vi "Wii_2D_mapping.vi"(0 "Wii_X_off":dbl, 5 "Wii_Y_off":dbl, 9 "previous_X":i32, 11 "previous_Y":i32, 13 "X_Y_speed":dbl) -> (4 "X":i32, 6 "Y":i32)   [LabVIEW 2011]
panel:
  out "X_resolution":i16
  out "Y_resolution":i16
  out "Ymax":i16
  out "Xmax":i16=2
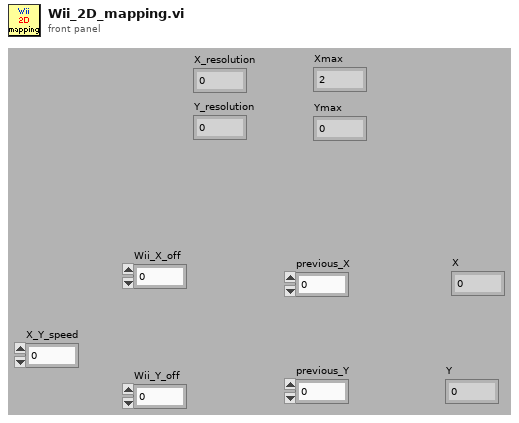
[diagram p1: front panel]
types:
  T1 = typedef "LVAllMonitorsDisplayTypeDef.ctl" = cluster{"Bounds":cluster{"Left":i16, "Top":i16, "Right":i16, "Bottom":i16}, "Depth":i16}[]
  T2 = cluster{"Bounds":cluster{"Left":i16, "Top":i16, "Right":i16, "Bottom":i16}, "Depth":i16}
  T3 = cluster{"Left":i16, "Top":i16, "Right":i16, "Bottom":i16}
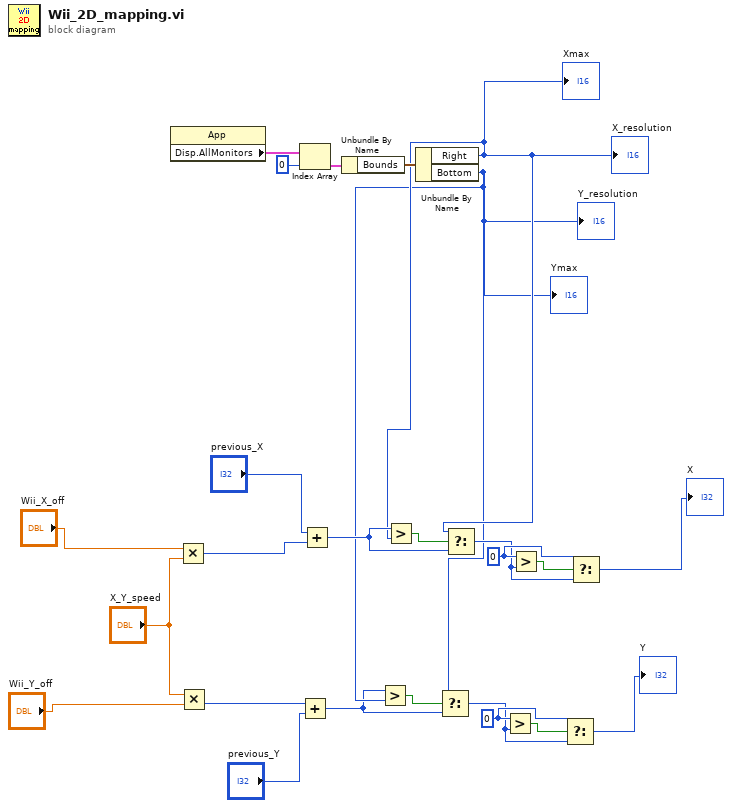
[diagram p0: block diagram]
diagram:
  w6 = i16 0 ("x")
  w10 = i16 0 ("x")
  n1 = property class="App"() -> ("Disp.AllMonitors"=w23:T1)  [unwired: 2 in, 2 out]
  n2 = Multiply(x="Wii_X_off", y="X_Y_speed") -> (x*y=w21:i32)
  n3 = Multiply(x="X_Y_speed", y="Wii_Y_off") -> (x*y=w19:i32)
  n4 = Index Array(array=w23, index=u16 0 ("Front Panel Window:Monitor")) -> (element=w25:T2)
  n5 = Add(x=w19, y="previous_Y") -> (x+y=w2:i32)
  n6 = Add(x="previous_X", y=w21) -> (x+y=w14:i32)
  n7 = Unbundle By Name(w25) -> ("Bounds"=w22:T3)
  n8 = Unbundle By Name(w22) -> ("Right"=w13:i16, "Bottom"=w3:i16)
  "Xmax" <- w13
  "Ymax" <- w3
  "Y_resolution" <- w3
  "X_resolution" <- w13
  n9 = Greater?(x=w2, y=w3) -> (0:w8:bool)
  n10 = Greater?(x=w14, y=w13) -> (0:w17:bool)
  n11 = Select(t=w3, s=w8, f=w2) -> (s? t:f=w5:i32)
  n12 = Select(t=w13, s=w17, f=w14) -> (s? t:f=w9:i32)
  n13 = Greater?(x=w6, y=w5) -> (0:w7:bool)
  n14 = Greater?(x=w10, y=w9) -> (0:w12:bool)
  n15 = Select(t=w6, s=w7, f=w5) -> (s? t:f=→"Y":i32)
  n16 = Select(t=w10, s=w12, f=w9) -> (s? t:f=→"X":i32)
